vi "FPGA Wait on IRQ(s).vi"   [LabVIEW 2010, in "FPGA Interface Base.lvclass"]
uses:
  <userlib>/_FPGA Interface Advanced Tools/FPGA Interface Base/FPGA Interface Base.lvclass
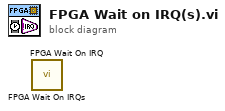
[diagram p0: block diagram]
diagram:
  n1 = call <userlib>:"FPGA Wait On IRQs.vi"() -> ()  [unwired: 8 in, 4 out]
  n2 = call <userlib>:"FPGA Wait On IRQ.vi"() -> ()  [unwired: 8 in, 4 out]
